vi "pot.vi"() -> ()   [LabVIEW 2025]
panel:
  out "2D Picture":picture
  in  "Port":dbl
  in  "Jetson IP Address":string
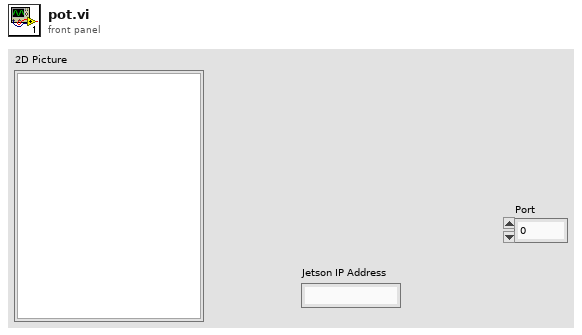
[diagram p1: front panel]
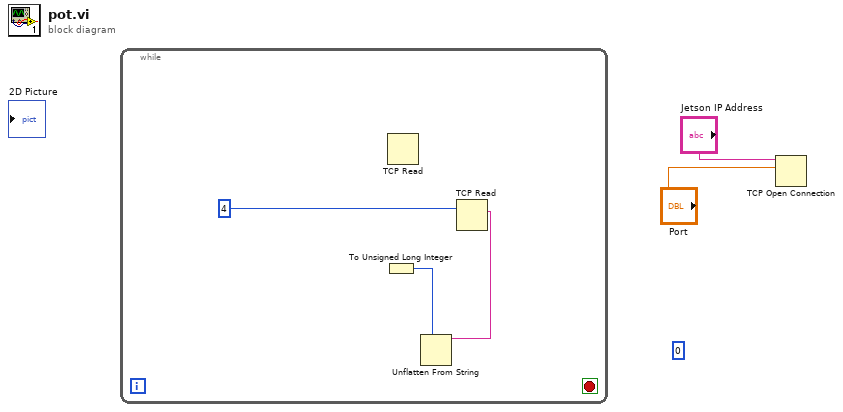
[diagram p0: block diagram]
diagram:
  (unwired) 0
  n1 = while {
    stop <- _ stop-if-true
    n2 = To Unsigned Long Integer() -> (unsigned 32bit integer=w5:u32)  [unwired: 1 in]
    n3 = TCP Read() -> ()  [unwired: 5 in, 3 out]
    n4 = TCP Read(bytes to read=4) -> (data out=w3:string)  [unwired: 4 in, 2 out]
    n5 = Unflatten From String(type=w5, binary string=w3) -> ()  [unwired: 3 in, 3 out]
  }
  n6 = TCP Open Connection(address="Jetson IP Address", remote port or service name="Port") -> ()  [unwired: 3 in, 2 out]
